vi "Actor Core.vi"(8 "error in":errorcluster, 11 "Actor in":refnum<class "Sensor & Control.lvclass">) -> (0 "error out":errorcluster, 3 "Actor out":refnum<class "Actor.lvclass">)   [LabVIEW 2013, in "Sensor & Control.lvib.lvlib" / "Sensor & Control.lvclass"]
doc: "This is Actor Core.vi, the main message handling loop for Actors. An actor usually just sits in this loop and processes messages as they arrive. Any error returned by the message Do.vi call will stop the loop, with error code 43 as the canonical signal to stop with no error sent to caller. Descendants may override that in Handle Error.vi."
uses:
  Sensor & Control.lvclass
  PluginInterface/Actor Framework.lvlibp/Actor/Actor.lvclass
  Sensor & Control.lvclass/Sensor & Control.ctl
  PluginInterface/PluginInterface.lvlibp/PluginInterfaceClass/PluginInterface.lvclass
  PluginInterface/Actor Framework.lvlibp/Message Enqueuer/Message Priority.ctl
  Write Graph.vi
  Write Setpoint.vi
  Write Value.vi
  Write Graph History.vi
  Write Sampling Interval.vi
  PluginInterface/PluginInterface.lvlibp/PluginInterfaceClass/Write VI Refnum.vi
  PluginInterface/Actor Framework.lvlibp/Message Enqueuer/Enqueue.vi
  Sensor & Control Messages/Initialize Msg/Initialize Msg.lvclass
  Sensor & Control Messages/Update Graphs Msg/Update Graphs Msg.lvclass
  Sensor & Control Messages/Update Setpoint Msg/Update Setpoint Msg.lvclass
  Sensor & Control Messages/Log Data Msg/Log Data Msg.lvclass
  Sensor & Control Messages/Write MFC Msg/Write Hardware Msg.lvclass
  Sensor & Control Messages/Read MFC Msg/Read Hardware Msg.lvclass
  PluginInterface/Actor Framework.lvlibp/Message Enqueuer/Message Enqueuer.lvclass
  PluginInterface/Actor Framework.lvlibp/Stop Msg/Stop Msg.lvclass
panel:
  in  "stop signal":bool
  in  "Sampling Interval":i32=5000
  in  "Round Color Box 2":u32(colorbox)=16728642
  in  "Round Color Box 1":u32(colorbox)=483491
  in  "Setpoint":dbl
  out "Value":dbl
  in  "Graph History":dbl=300.0
  out "Graph":T1(graph)
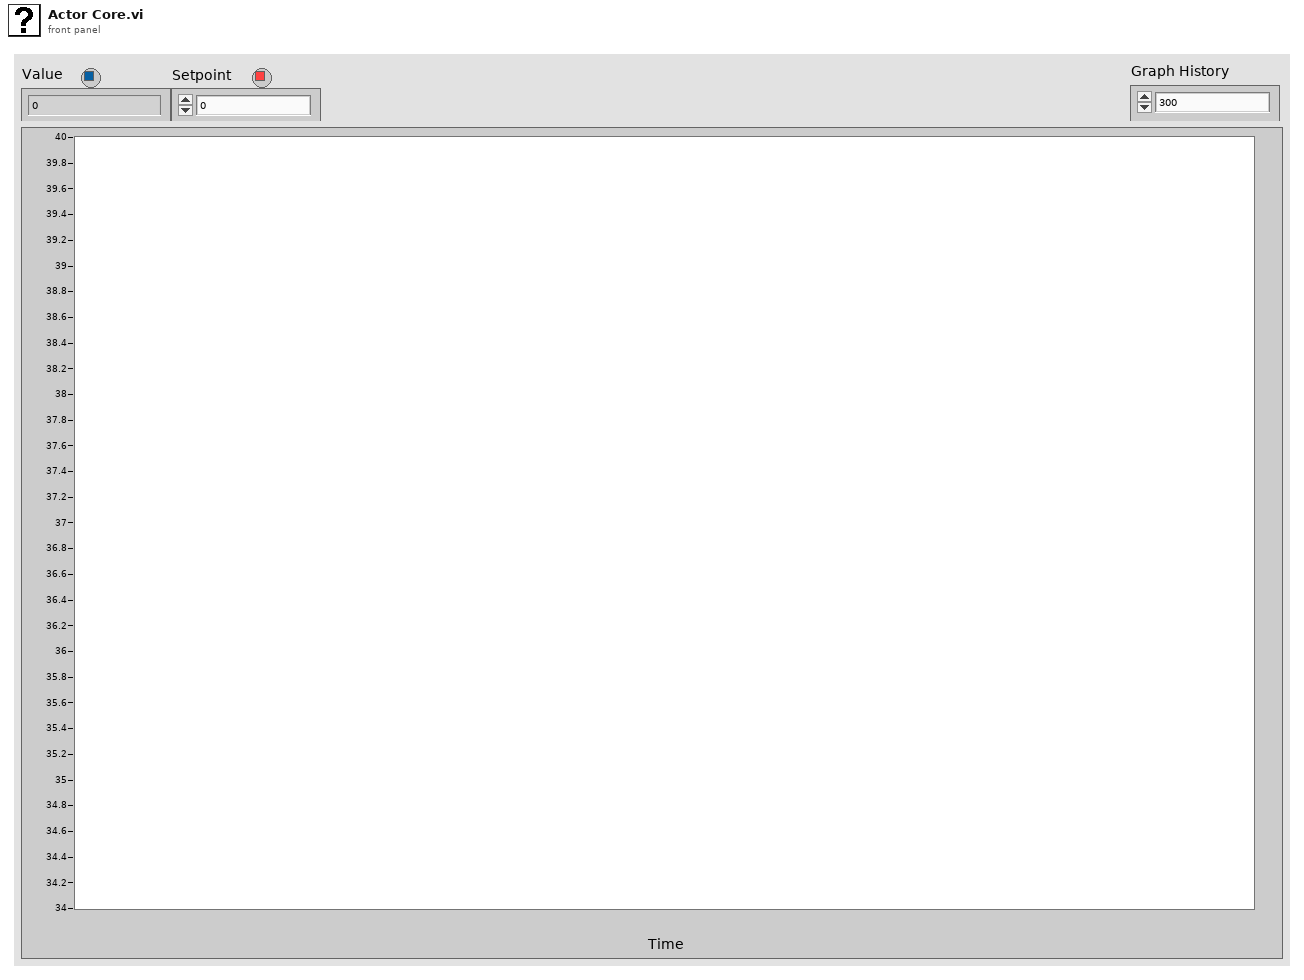
[diagram p1: front panel]
types:
  T1 = cluster{"output array":dbl[], "output array":dbl[]}[]
  T2 = typedef "Actor Framework.lvlibp/Message Enqueuer.lvclass/Message Priority.ctl" = enum16{"Low", "Normal", "High"}
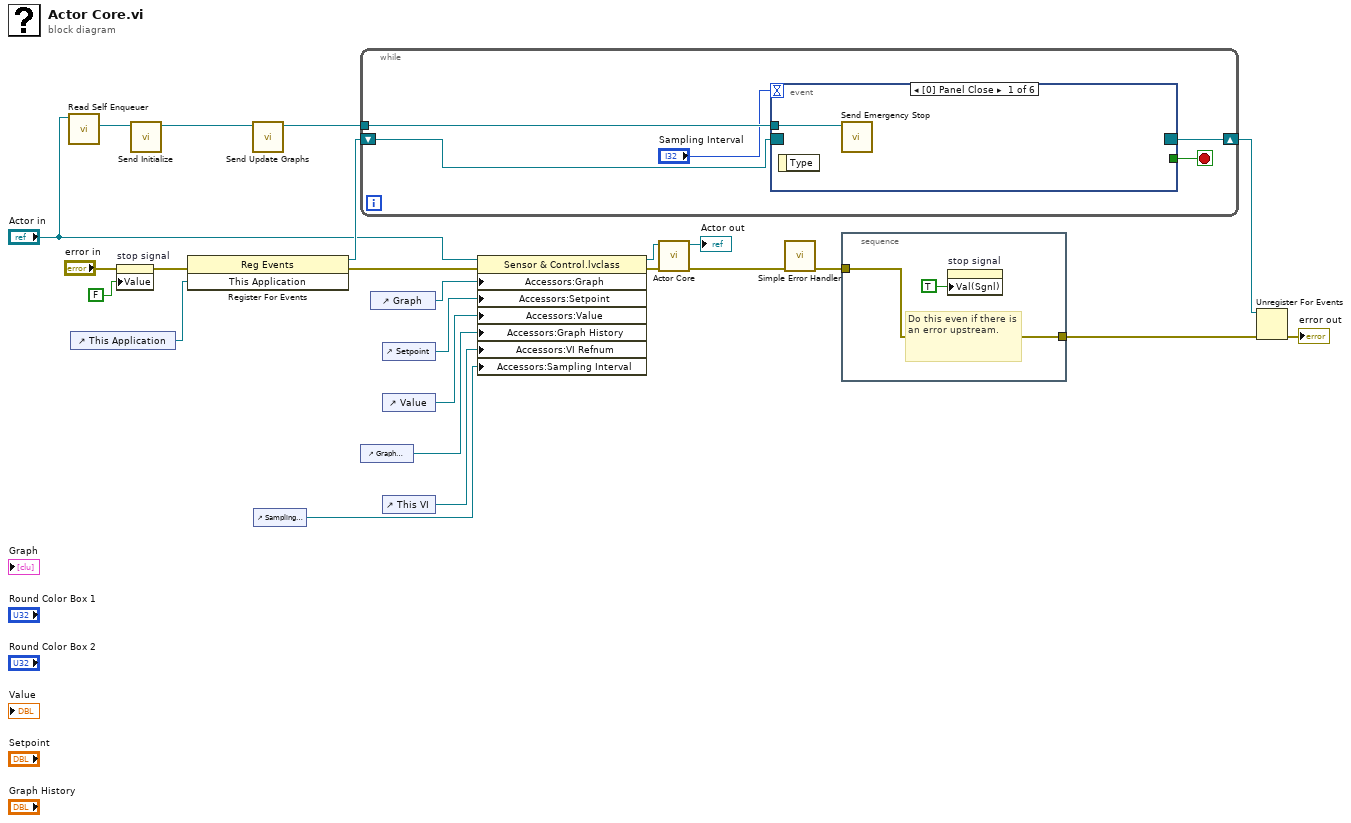
[diagram p0: block diagram]
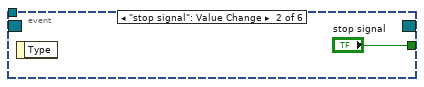
[diagram p2: hidden frame]
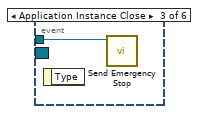
[diagram p3: hidden frame]
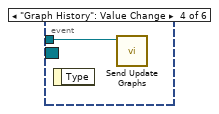
[diagram p4: hidden frame]
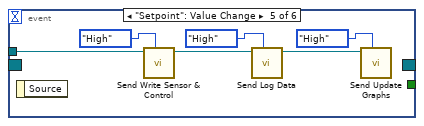
[diagram p5: hidden frame]
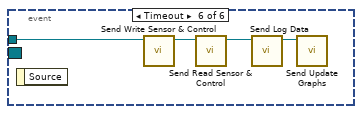
[diagram p6: hidden frame]
diagram:
  n1 = call "Read Self Enqueuer.vi"("Actor"="Actor in") -> ("Self Enqueuer"=w6:refnum<class "Message Enqueuer.lvclass">)  [unwired: 10 in]
  n2 = control-ref of="This Application"() -> (w17:refnum<vi>)
  n3 = property on="stop signal" class="Bool (strict)"(error in="error in", "Value"=FALSE ("stop")) -> (error out=w18:errorcluster)  [unwired: 1 in, 1 out]
  n4 = call "Send Initialize.vi"("Message Enqueuer"=w6) -> ("Message Enqueuer out"=w3:refnum<class "Message Enqueuer.lvclass">)  [unwired: 9 in, 1 out]
  n5 = register-events(error in=w18, w17) -> (reference out=w21:refnum<event-registration>, error out=w5:errorcluster)  [unwired: 1 in]
  n6 = call "Send Update Graphs.vi"("Message Enqueuer"=w3) -> ("Message Enqueuer out"=w2:refnum<class "Message Enqueuer.lvclass">)  [unwired: 9 in, 1 out]
  n7 = control-ref of="Sampling Interval"() -> (w1:refnum<vi>)
  n8 = while {
    tunnel: w2 -> [w29]
    shift-right: [w26] -> w20
    shift-left: w21 -> [w27]
    stop <- w28 stop-if-true
    n9 = event shown="[0] Panel Close" {
      selector: w27 -> [_ _ _ _ _ _]
      dyn-events: [_ _ _ _ _ _] -> w26
      timeout: "Sampling Interval" -> [_ _ _ _ _ _]
      tunnel: w29 -> [w30 _ w32 w33 w39 w43]
      tunnel: [_ "stop signal" _ _ _ _] -> w28
      event Panel Close {
        n10 = event-data() -> ()  [unwired: 1 in, 1 out]
        n11 = call "Send Emergency Stop.vi"("Message Enqueuer"=w30) -> ()  [unwired: 10 in, 1 out]
      }
      event "stop signal": Value Change {
        n12 = event-data() -> ()  [unwired: 1 in, 1 out]
      }
      event Application Instance Close {
        n13 = event-data() -> ()  [unwired: 1 in, 1 out]
        n14 = call "Send Emergency Stop.vi"("Message Enqueuer"=w32) -> ()  [unwired: 10 in, 1 out]
      }
      event "Graph History": Value Change {
        n15 = event-data() -> ()  [unwired: 1 in, 1 out]
        n16 = call "Send Update Graphs.vi"("Message Enqueuer"=w33) -> ()  [unwired: 9 in, 2 out]
      }
      event "Setpoint": Value Change {
        n17 = event-data() -> ()  [unwired: 1 in, 1 out]
        n18 = call "Send Write Sensor & Control.vi"("Message Priority (Normal)"=Message_Priority."High", "Message Enqueuer"=w39) -> ("Message Enqueuer out"=w35:refnum<class "Message Enqueuer.lvclass">)  [unwired: 8 in, 1 out]
        n19 = call "Send Log Data.vi"("Message Priority (Normal)"=Message_Priority."High", "Message Enqueuer"=w35) -> ("Message Enqueuer out"=w34:refnum<class "Message Enqueuer.lvclass">)  [unwired: 8 in, 1 out]
        n20 = call "Send Update Graphs.vi"("Message Priority (Normal)"=Message_Priority."High", "Message Enqueuer"=w34) -> ()  [unwired: 8 in, 2 out]
      }
      event Timeout {
        n21 = event-data() -> ()  [unwired: 1 in, 1 out]
        n22 = call "Send Write Sensor & Control.vi"("Message Enqueuer"=w43) -> ("Message Enqueuer out"=w40:refnum<class "Message Enqueuer.lvclass">)  [unwired: 9 in, 1 out]
        n23 = call "Send Read Sensor & Control.vi"("Message Enqueuer"=w40) -> ("Message Enqueuer out"=w42:refnum<class "Message Enqueuer.lvclass">)  [unwired: 9 in, 1 out]
        n24 = call "Send Log Data.vi"("Message Enqueuer"=w42) -> ("Message Enqueuer out"=w41:refnum<class "Message Enqueuer.lvclass">)  [unwired: 9 in, 1 out]
        n25 = call "Send Update Graphs.vi"("Message Enqueuer"=w41) -> ()  [unwired: 9 in, 2 out]
      }
    }
  }
  n26 = control-ref of="Graph History"() -> (w8:refnum<vi>)
  n27 = control-ref of="Graph"() -> (w7:refnum<vi>)
  n28 = control-ref of="Setpoint"() -> (w10:refnum<vi>)
  n29 = control-ref of="Value"() -> (w11:refnum<vi>)
  n30 = control-ref of="This VI"() -> (w4:refnum<vi>)
  n31 = property class="Sensor & Control.lvclass"(reference="Actor in", error in=w5, "Accessors:Graph"=w7, "Accessors:Setpoint"=w10, "Accessors:Value"=w11, "Accessors:Graph History"=w8, "Accessors:VI Refnum"=w4, "Accessors:Sampling Interval"=w1) -> (reference out=w16:refnum<class "Sensor & Control.lvclass">, error out=w12:errorcluster)
  n32 = call-parent "Actor Core.vi"("error in"=w12, "Actor in"=w16) -> ("error out"=w23:errorcluster, "Actor out"=→"Actor out":refnum<class "Actor.lvclass">)  [unwired: 8 in]
  n33 = call <vilib>:"Simple Error Handler.vi"("error in (no error)"=w23) -> ("error out"=w22:errorcluster)  [unwired: 4 in, 4 out]
  n34 = stacked-sequence {
    tunnel: [w44] -> w19
    tunnel: w22 -> [w44]
    frame #0 {
      # "Do this even if there is an error upstream."
      n35 = property on="stop signal" class="Bool (strict)"("Val(Sgnl)"=TRUE ("stop")) -> ()  [unwired: 2 in, 2 out]
    }
  }
  n36 = Unregister For Events(event registration refnum=w20, error in=w19) -> (error out=→"error out":errorcluster)
